vi "Pause Command.vi"(8 "error in":errorcluster, 11 "CoreOOB_Rx in":refnum<class "CIFTemplateCoreOOB_Rx.lvclass">) -> (0 "error out":errorcluster, 3 "CoreOOB_Rx out":refnum<class "CIFTemplateCoreOOB_Rx.lvclass">)   [LabVIEW 2021, in "CIFTemplateCoreOOB_Rx.lvclass"]
uses:
  CIFTemplateCoreOOB_Rx.lvclass
  D:/dev/CIF-Core-LabVIEW/src/CIF_Utilities/CifOutOfBand/CIFOutOfBand.lvclass
  Typedef/OOB Core Commands.ctl
  CIFUtilities/CifOutOfBand/CIFOutOfBand.lvclass/CIFOutOfBand.ctl
  CIFUtilities/CifOutOfBand/CIFOutOfBand.lvclass
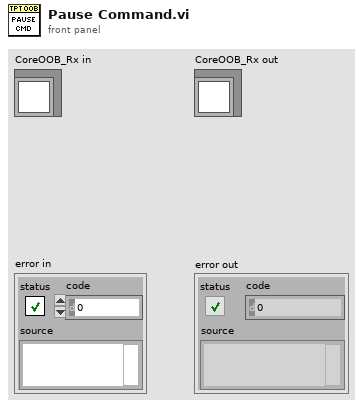
[diagram p1: front panel]
types:
  T1 = typedef "CIFTemplateCoreOOB_Rx.lvclass/OOB Core Commands.ctl" = enum8{"Start", "StartFTE", "Pause", "Stop", "Restart", "RestartFTE", "RefreshStats", "UpdateConfig"}
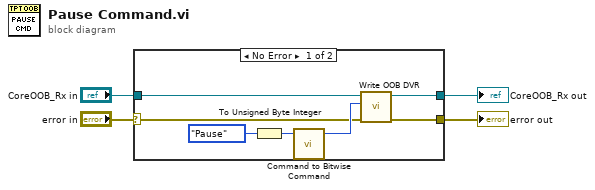
[diagram p0: block diagram]
diagram:
  n1 = case shown="No Error" "error in" {
    selector: "error in" -> [w5 w13]
    tunnel: [w10 w13] -> w3
    tunnel: "CoreOOB_Rx in" -> [w6 w12]
    tunnel: [w11 w12] -> w1
    frame No Error {
      n2 = To Unsigned Byte Integer(number=OOB_Core_Commands."Pause" ("OOB Main Commands")) -> (unsigned 8bit integer=w8:u8)
      n3 = call "Command to Bitwise Command.vi"("OOB Command"=w8) -> ("bit command"=w7:u64)  [unwired: 3 in]
      n4 = call "Write OOB DVR.vi"("error in"=w5, "Commands (bitwise)"=w7, "OOB in"=w6) -> ("error out"=w10:errorcluster, "OOB out"=w11:refnum<class "CIFTemplateCoreOOB_Rx.lvclass">)  [unwired: 7 in]
    }
    frame Error {
    }
  }
  "error out" <- w3
  "CoreOOB_Rx out" <- w1
